vi "Read Data from HW.vi"(11 "Custom Device in":refnum<class "SystemMonitor Engine.lvclass">) -> (0 "error out":errorcluster, 3 "Custom Device out":refnum<class "SystemMonitor Engine.lvclass">)   [LabVIEW 2026, in "SystemMonitor Engine.lvlib" / "SystemMonitor Engine.lvclass"]
uses:
  SystemMonitor Engine.lvclass
  SystemMonitor Engine.lvclass/SystemMonitor Engine.ctl
  <userlib>/NIVS Inline Async API (Express)/_VS Inline Async API (Express)/VS Inline Async API (Express)/VS Inline Async API (Express).lvclass/VS Inline Async API (Express).ctl
  <userlib>/NIVS Inline Async API (Express)/_Data Access Engine (Express)/Data Access Engine (Express)/Data Access Engine (Express).lvclass/Data Access Engine (Express).ctl
  <userlib>/NIVS Inline Async API (Express)/_Data Access Engine (Express)/Access Type Classes/Write/Write.lvclass/Write.ctl
  <userlib>/NIVS Inline Async API (Express)/_Data Access Engine (Express)/Access Type Classes/ReadWrite/ReadWrite.lvclass/ReadWrite.ctl
  <userlib>/NIVS Inline Async API (Express)/_VS Inline Async API (Express)/Error Handling Process/SubVIs/Error.GetError.vi
  <userlib>/NIVS Inline Async API (Express)/_Data Access Engine (Express)/Access Type Classes/ReadWrite/ReadWrite.EngineData.vi
  <userlib>/NIVS Inline Async API (Express)/_Data Access Engine (Express)/Access Type Classes/Write/Write.EngineData.vi
  <userlib>/Custom Device Interfaces_v1.lvlibp/CustomDeviceAPI/Custom Device API.lvclass
  <userlib>/NIVS Inline Async API (Express)/_VS Inline Async API (Express)/VS Inline Async API (Express)/VS Inline Async API (Express).lvclass
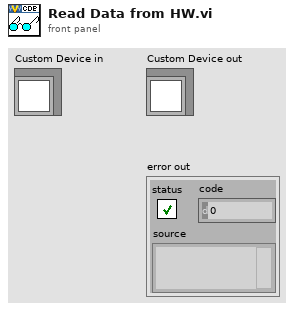
[diagram p1: front panel]
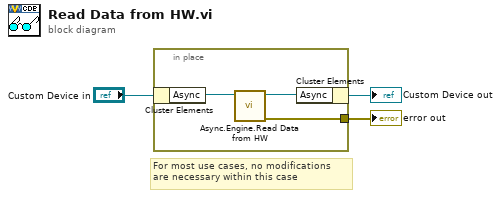
[diagram p0: block diagram]
diagram:
  # "For most use cases, no modifications \nare necessary within this case"
  n1 = in-place {
    in-place-border: [w4] -> w3
    n2 = in-place-cluster #1("Custom Device in") -> ("Async"=w6:refnum<class "VS Inline Async API (Express).lvclass">)
    n3 = call <userlib>:"Async.Engine.Read Data from HW.vi"("Async in"=w6) -> ("error out"=w4:errorcluster, "Async out"=w5:refnum<class "VS Inline Async API (Express).lvclass">)  [unwired: 9 in]
    n4 = in-place-cluster #1("Async"=w5) -> (→"Custom Device out":refnum<class "SystemMonitor Engine.lvclass">)
  }
  "error out" <- w3
